vi "试剂余量显示UI.vi"() -> ()   [LabVIEW 2016, in "斯坦道氟化物.lvlib"]
uses:
  <vilib>/Utility/miscctls.llb/LVPointTypeDef.ctl
panel:
  in  "余量 14":string
  in  "余量 13":string
  in  "余量 12":string
  in  "余量 11":string
  in  "余量 10":string
  in  "余量 9":string
  in  "余量 8":string
  in  "余量 7":string
  in  "余量 6":string
  in  "余量 5":string
  in  "余量 4":string
  in  "余量 3":string
  in  "余量 2":string
  in  "余量":string
  in  "关闭":bool
  in  "全部重置":bool
  in  "试剂容量设置":bool
  in  "试剂名称设置":bool
  in  "重置 14":bool
  out "试剂 14":dbl(slide) caption="V9-2.试剂14" scale=0.0..100.0 scale format="%#_f %%"
  in  "重置 13":bool
  out "试剂 13":dbl(slide) caption="V9-1.试剂13" scale=0.0..100.0 scale format="%#_f %%"
  in  "重置 12":bool
  out "试剂 12":dbl(slide) caption="V12.试剂12" scale=0.0..100.0 scale format="%#_f %%"
  in  "重置 11":bool
  out "试剂 11":dbl(slide) caption="V11.试剂11" scale=0.0..100.0 scale format="%#_f %%"
  in  "重置 10":bool
  out "试剂 10":dbl(slide) caption="V10.试剂10" scale=0.0..100.0 scale format="%#_f %%"
  in  "重置 9":bool
  out "试剂 9":dbl(slide) caption="V9.试剂9" scale=0.0..100.0 scale format="%#_f %%"
  in  "重置 8":bool
  out "试剂 8":dbl(slide) caption="V8.试剂8" scale=0.0..100.0 scale format="%#_f %%"
  in  "重置 7":bool
  out "试剂 7":dbl(slide) caption="V7.试剂7" scale=0.0..100.0 scale format="%#_f %%"
  in  "重置 6":bool
  out "试剂 6":dbl(slide) caption="V6.试剂6" scale=0.0..100.0 scale format="%#_f %%"
  in  "重置 5":bool
  out "试剂 5":dbl(slide) caption="V5.试剂5" scale=0.0..100.0 scale format="%#_f %%"
  in  "重置 4":bool
  out "试剂 4":dbl(slide) caption="V4.试剂4" scale=0.0..100.0 scale format="%#_f %%"
  in  "重置 3":bool
  out "试剂 3":dbl(slide) caption="V3.试剂3" scale=0.0..100.0 scale format="%#_f %%"
  in  "重置 2":bool
  out "试剂 2":dbl(slide) caption="V2.试剂2" scale=0.0..100.0 scale format="%#_f %%"
  in  "重置":bool
  out "试剂":dbl(slide) caption="V1.试剂1" scale=0.0..100.0 scale format="%#_f %%"
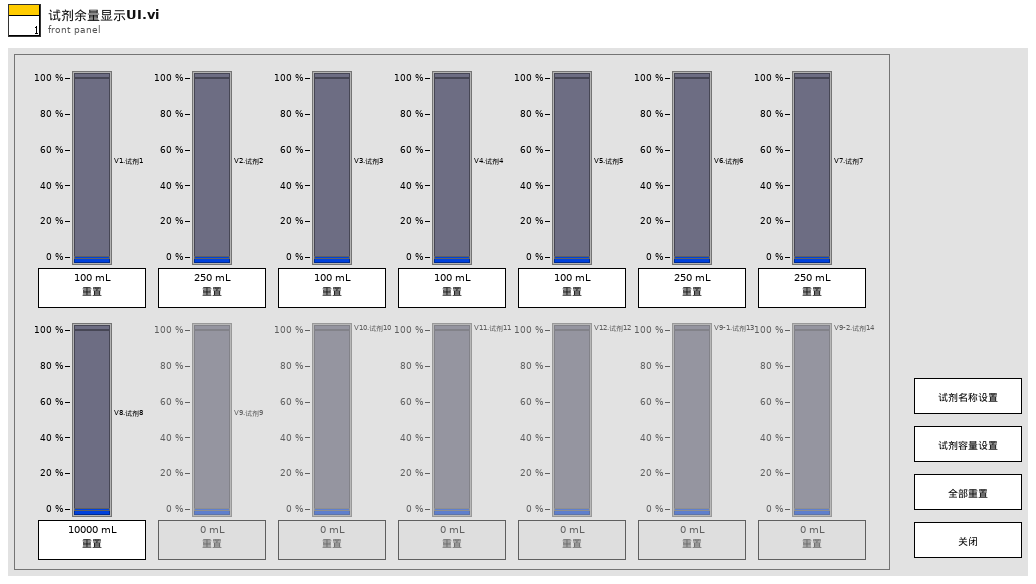
[diagram p1: front panel]
types:
  T1 = typedef "LVPointTypeDef.ctl" = cluster{"Horizontal":i16, "Vertical":i16}
  T2 = enum8{"Enabled", "Disabled", "Disabled and Grayed Out"}
  T3 = cluster{"时间标识":timestamp, "设备":string, "日志信息":string, "流程参数":string}
  T4 = cluster{"V1":sgl, "V2":sgl, "V3":sgl, "V4":sgl, "V5":sgl, "V6":sgl, "V7":sgl, "V8":sgl, "V9":sgl, "V10":sgl, "V11":sgl, "V12":sgl, "V9-1":sgl, "V9-2":sgl}
  T5 = cluster{"V":string, "V 2":string, "V 3":string, "V 4":string, "V 5":string, "V 6":string, "V 7":string, "V 8":string, "V 9":string, "V 10":string, "V 11":string, "V 12":string, "V9-1":string, "V9-2":string}
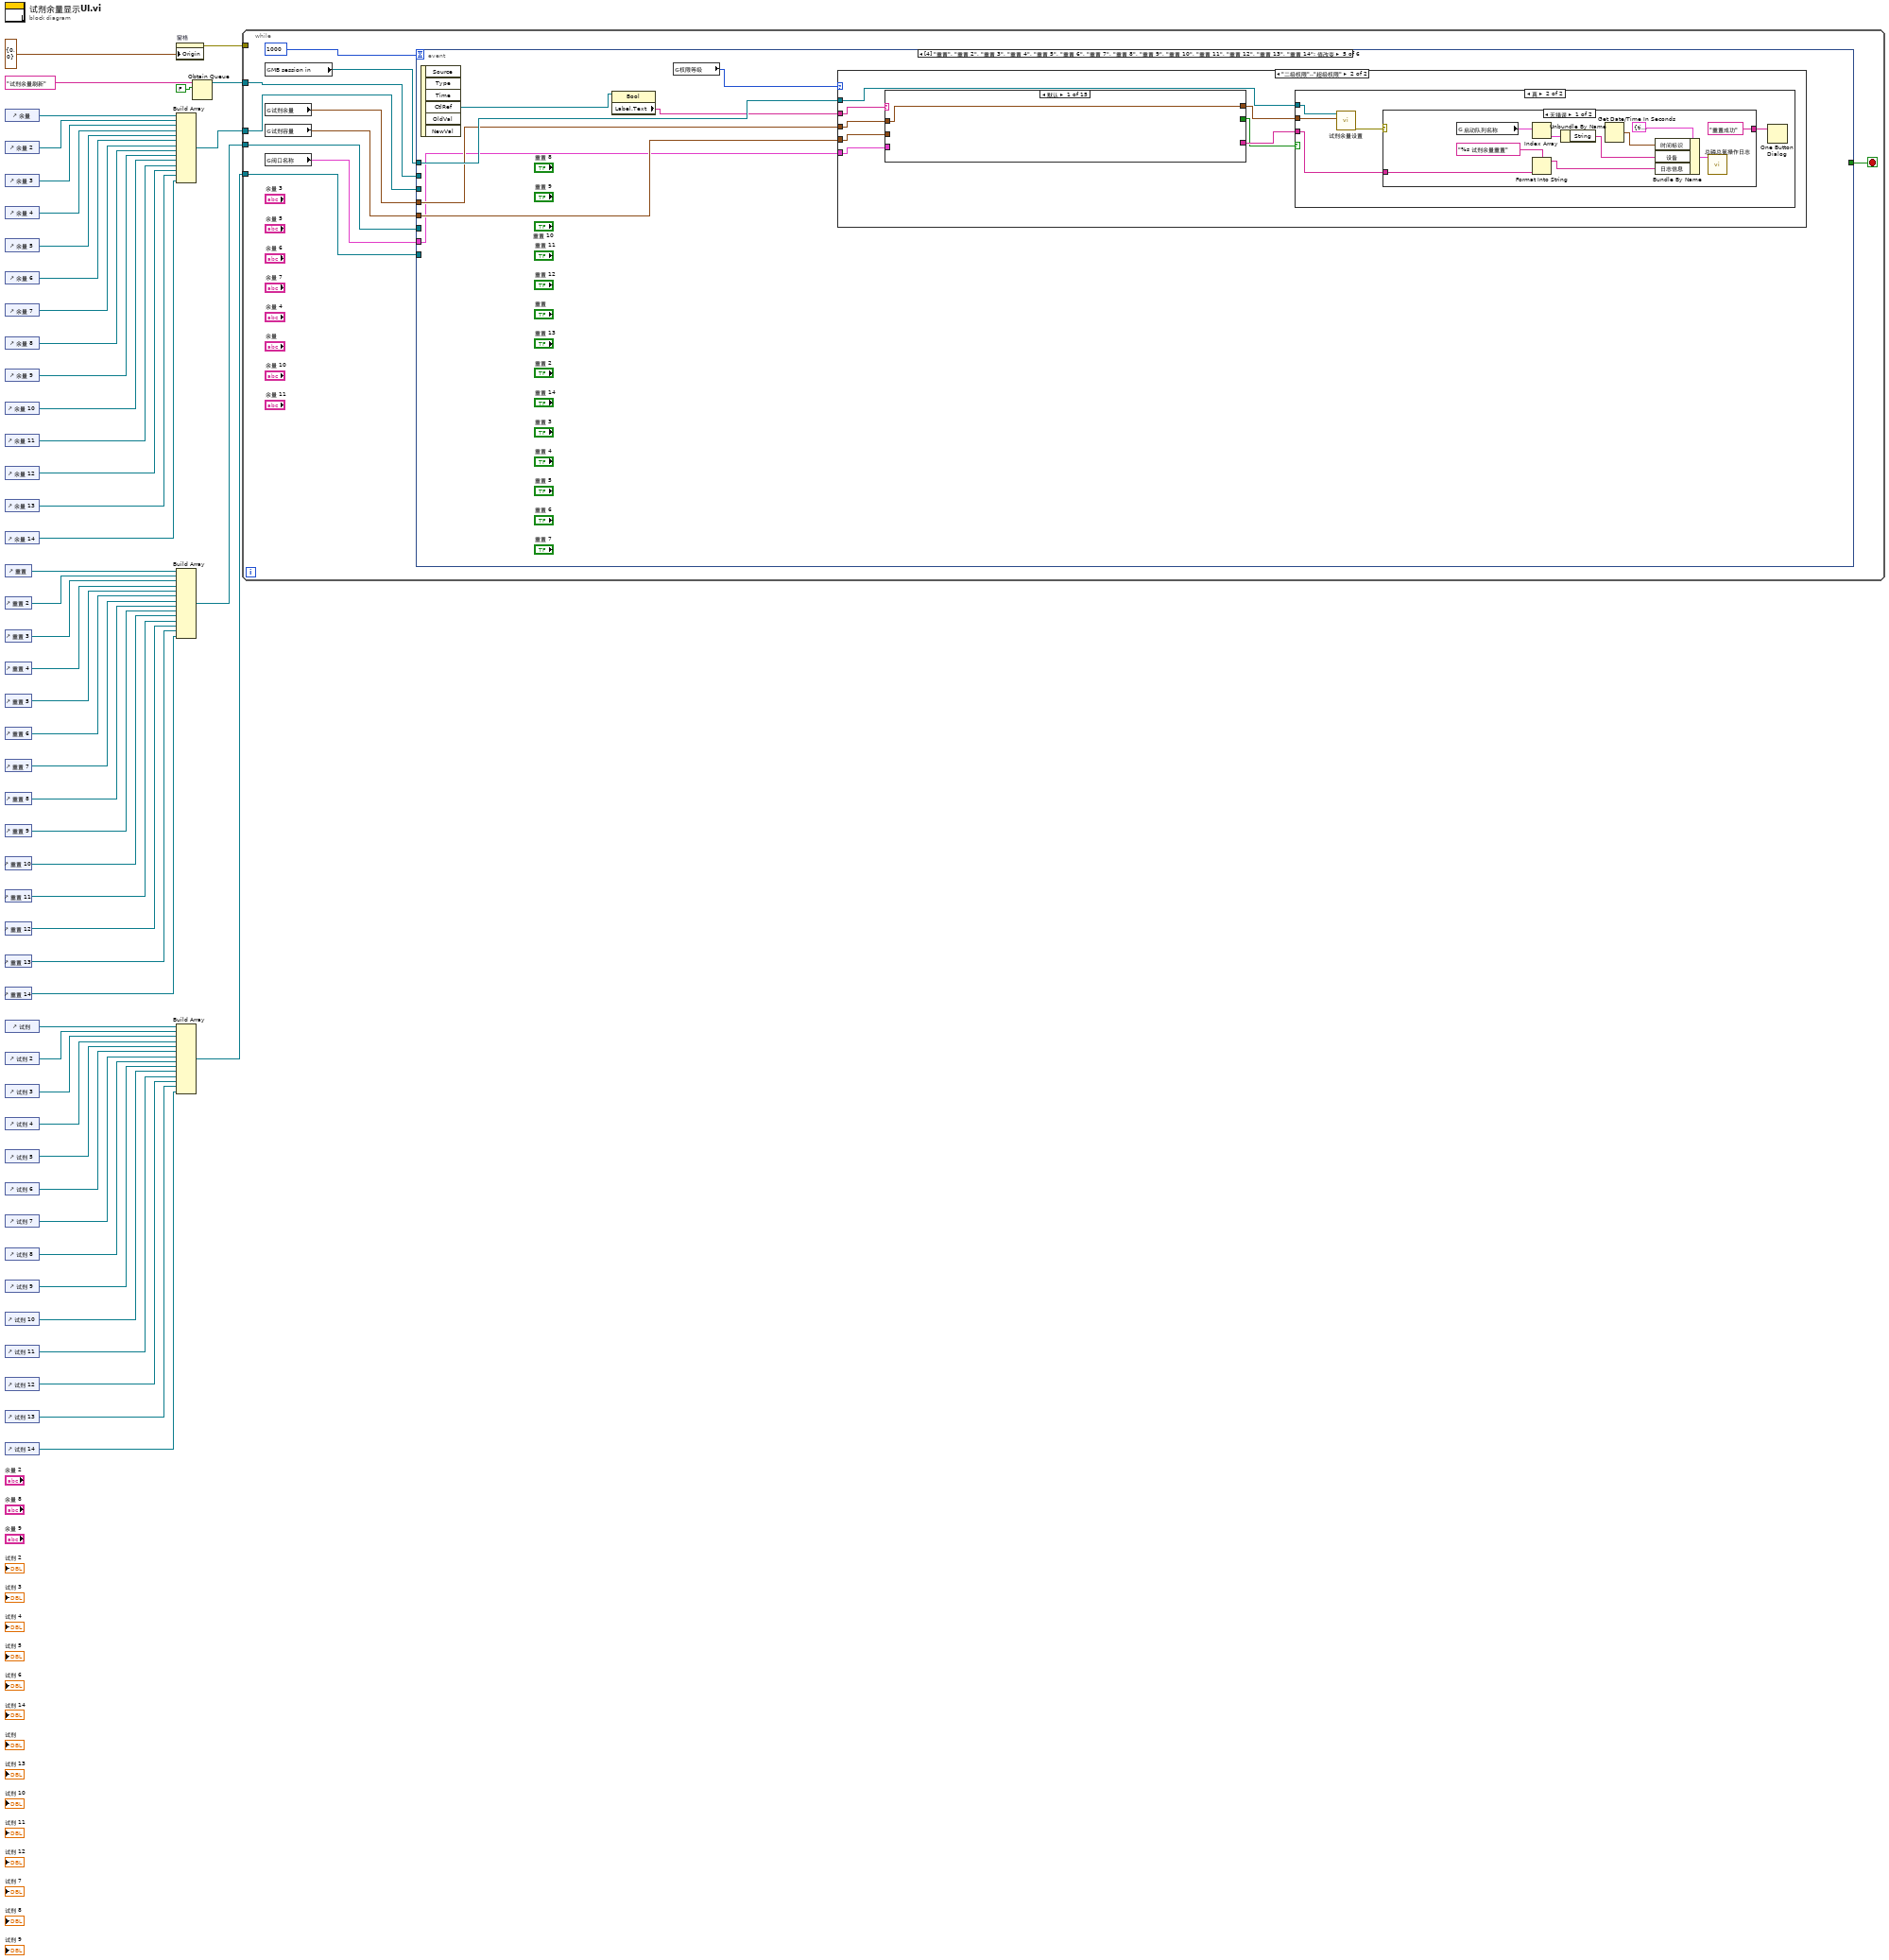
[diagram p0: block diagram]
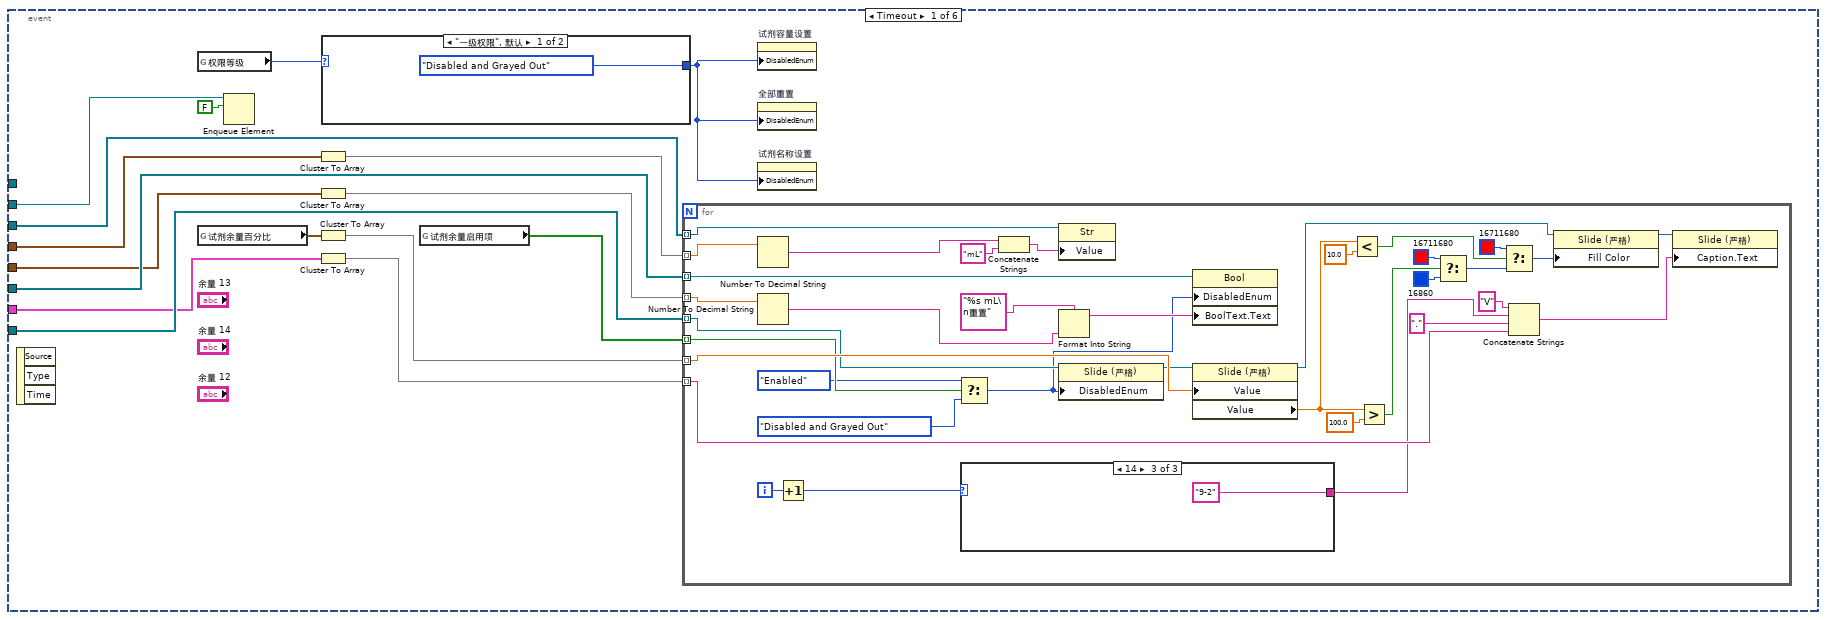
[diagram p2: hidden frame]
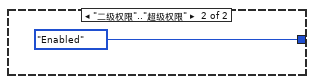
[diagram p3: hidden frame]
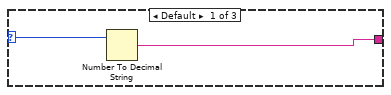
[diagram p4: hidden frame]
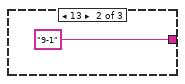
[diagram p5: hidden frame]
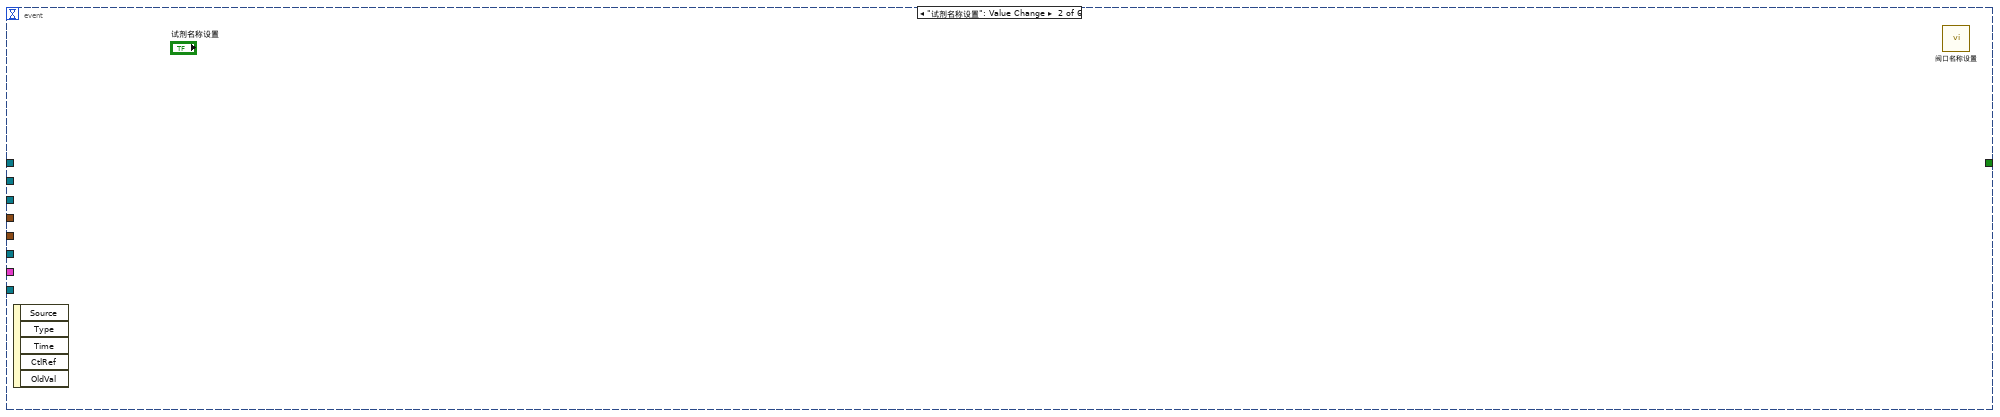
[diagram p6: hidden frame]
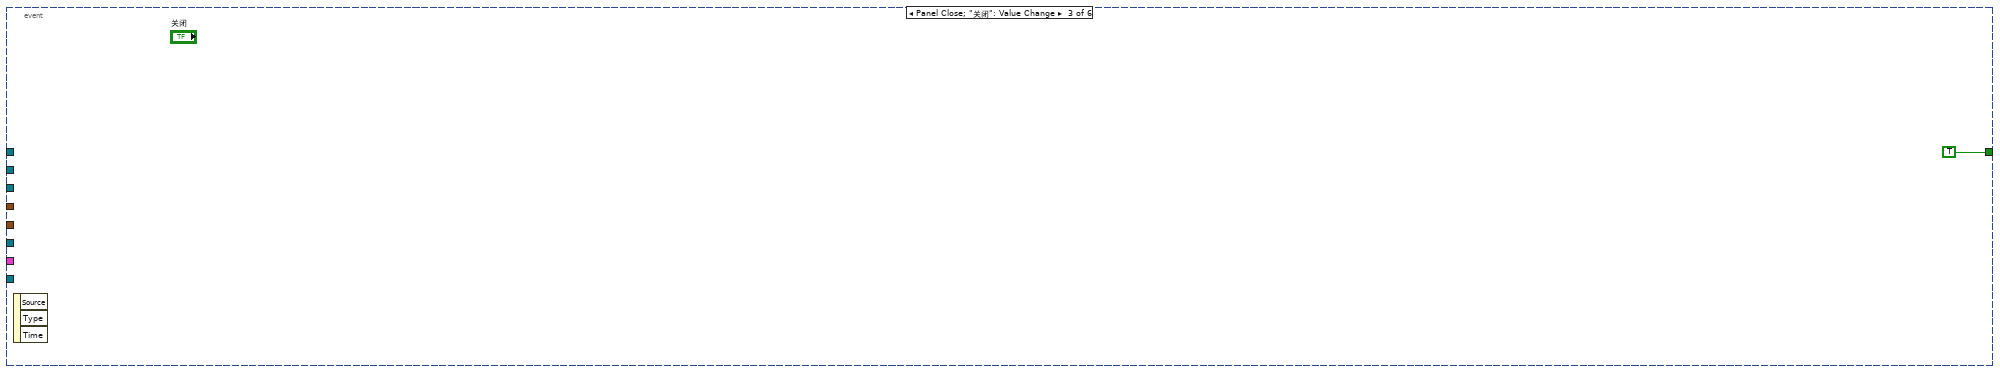
[diagram p7: hidden frame]
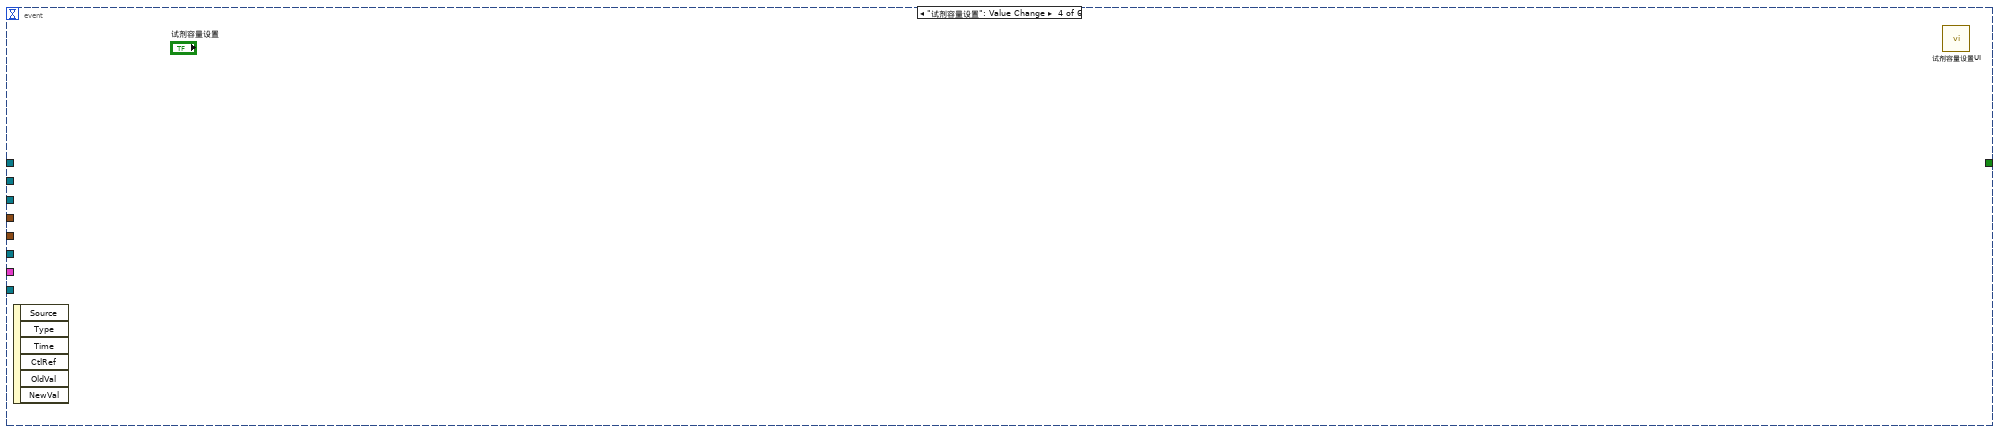
[diagram p8: hidden frame]
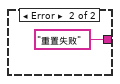
[diagram p11: hidden frame]
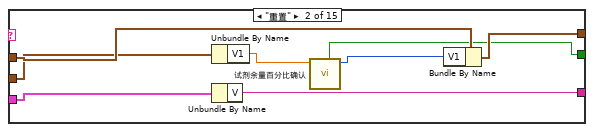
[diagram p12: hidden frame]
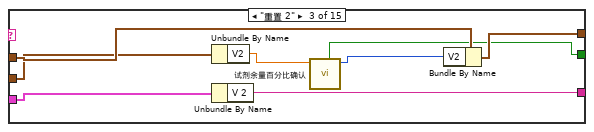
[diagram p13: hidden frame]
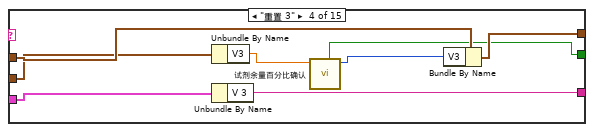
[diagram p14: hidden frame]
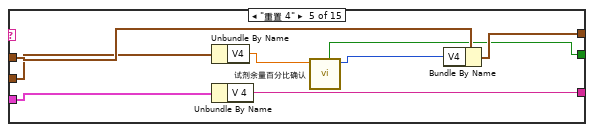
[diagram p15: hidden frame]
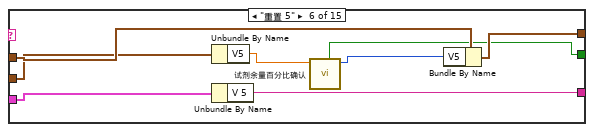
[diagram p16: hidden frame]
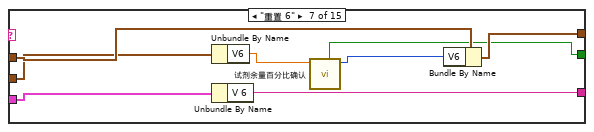
[diagram p17: hidden frame]
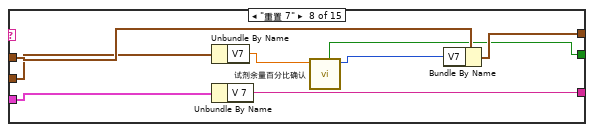
[diagram p18: hidden frame]
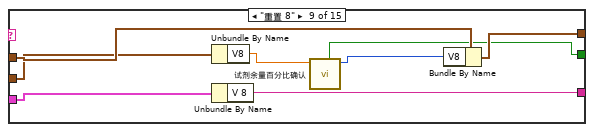
[diagram p19: hidden frame]
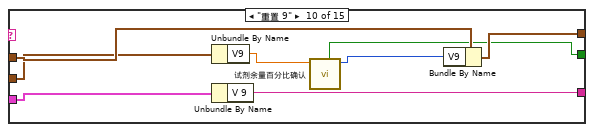
[diagram p20: hidden frame]
diagram:
  n1 = control-ref of="余量"() -> (w5:refnum<vi>)
  n2 = control-ref of="余量 2"() -> (w6:refnum<vi>)
  n3 = control-ref of="余量 3"() -> (w7:refnum<vi>)
  n4 = control-ref of="余量 4"() -> (w8:refnum<vi>)
  n5 = control-ref of="余量 5"() -> (w9:refnum<vi>)
  n6 = control-ref of="余量 6"() -> (w10:refnum<vi>)
  n7 = control-ref of="余量 7"() -> (w11:refnum<vi>)
  n8 = control-ref of="余量 8"() -> (w12:refnum<vi>)
  n9 = control-ref of="余量 9"() -> (w13:refnum<vi>)
  n10 = control-ref of="余量 10"() -> (w14:refnum<vi>)
  n11 = control-ref of="余量 11"() -> (w15:refnum<vi>)
  n12 = control-ref of="余量 12"() -> (w16:refnum<vi>)
  n13 = control-ref of="余量 13"() -> (w17:refnum<vi>)
  n14 = control-ref of="余量 14"() -> (w18:refnum<vi>)
  n15 = control-ref of="重置"() -> (w33:refnum<vi>)
  n16 = control-ref of="重置 2"() -> (w32:refnum<vi>)
  n17 = control-ref of="重置 3"() -> (w31:refnum<vi>)
  n18 = control-ref of="重置 4"() -> (w30:refnum<vi>)
  n19 = control-ref of="重置 5"() -> (w29:refnum<vi>)
  n20 = control-ref of="重置 6"() -> (w28:refnum<vi>)
  n21 = control-ref of="重置 7"() -> (w27:refnum<vi>)
  n22 = control-ref of="重置 8"() -> (w26:refnum<vi>)
  n23 = control-ref of="重置 9"() -> (w25:refnum<vi>)
  n24 = control-ref of="重置 10"() -> (w24:refnum<vi>)
  n25 = control-ref of="重置 11"() -> (w23:refnum<vi>)
  n26 = control-ref of="重置 12"() -> (w22:refnum<vi>)
  n27 = control-ref of="重置 13"() -> (w21:refnum<vi>)
  n28 = control-ref of="重置 14"() -> (w20:refnum<vi>)
  n29 = control-ref of="试剂"() -> (w50:refnum<vi>)
  n30 = control-ref of="试剂 2"() -> (w49:refnum<vi>)
  n31 = control-ref of="试剂 3"() -> (w48:refnum<vi>)
  n32 = control-ref of="试剂 4"() -> (w47:refnum<vi>)
  n33 = control-ref of="试剂 5"() -> (w46:refnum<vi>)
  n34 = control-ref of="试剂 6"() -> (w45:refnum<vi>)
  n35 = control-ref of="试剂 7"() -> (w44:refnum<vi>)
  n36 = control-ref of="试剂 8"() -> (w43:refnum<vi>)
  n37 = control-ref of="试剂 9"() -> (w42:refnum<vi>)
  n38 = control-ref of="试剂 10"() -> (w41:refnum<vi>)
  n39 = control-ref of="试剂 11"() -> (w40:refnum<vi>)
  n40 = control-ref of="试剂 12"() -> (w39:refnum<vi>)
  n41 = control-ref of="试剂 13"() -> (w38:refnum<vi>)
  n42 = control-ref of="试剂 14"() -> (w37:refnum<vi>)
  n43 = property on="窗格" class="Pane"("Origin"=T1 {"Horizontal"=0, "Vertical"=0} ("原点")) -> (error out=w34:errorcluster)  [unwired: 2 in, 1 out]
  n44 = Build Array(w5, w6, w7, w8, w9, w10, w11, w12, w13, w14, w15, w16, w17, w18) -> (w4:refnum<vi>[])
  n45 = Build Array(w33, w32, w31, w30, w29, w28, w27, w26, w25, w24, w23, w22, w21, w20) -> (w19:refnum<vi>[])
  n46 = Build Array(w50, w49, w48, w47, w46, w45, w44, w43, w42, w41, w40, w39, w38, w37) -> (w36:refnum<vi>[])
  n47 = Obtain Queue(name (unnamed)="试剂余量刷新" ("名称（未命名）"), element data type=FALSE) -> (queue out=w1:refnum<queue>)  [unwired: 3 in, 2 out]
  n48 = while {
    tunnel: w36 -> [w60]
    tunnel: w34 -> [_]
    tunnel: w19 -> [w59]
    tunnel: w4 -> [w55]
    tunnel: w1 -> [w51]
    stop <- w58 stop-if-true
    n49 = global read "VAR总磷总氮全局变量.vi" "MB session in"() -> (w56:refnum<class "MB_Master.lvclass">)
    n50 = global read "VAR总磷总氮全局变量.vi" "试剂余量"() -> (w53:T4)
    n51 = global read "VAR总磷总氮全局变量.vi" "试剂容量"() -> (w54:T4)
    n52 = global read "总磷总氮断电保存全局变量.vi" "阀口名称"() -> (w52:T5)
    n53 = event shown="[4] \"重置\", \"重置 2\", \"重置 3\", \"重置 4\", \"重置 5\", \"重置 6\", \"重置 7\", \"重置 8\", \"重置 9\", \"重置 10\", \"重置 11\", \"重置 12\", \"重置 13\", \"重置 14\": 值改变" {
      selector: _ -> [_ _ _ _ _ _]
      dyn-events: _ -> [_ _ _ _ _ _]
      timeout: 1000 -> [_ _ _ _ _ _]
      tunnel: w60 -> [w76 _ _ _ _ _]
      tunnel: w59 -> [w73 _ _ _ _ _]
      tunnel: [_ _ TRUE _ _ _] -> w58
      tunnel: w54 -> [w67 _ _ _ w122 _]
      tunnel: w53 -> [w66 _ _ _ w125 _]
      tunnel: w56 -> [_ _ _ _ w126 w265]
      tunnel: w55 -> [w70 _ _ _ _ _]
      tunnel: w52 -> [w63 _ _ _ w120 _]
      tunnel: w51 -> [w62 _ _ _ _ _]
      event Timeout {
        n54 = event-data() -> ()  [unwired: 1 in, 3 out]
        n55 = global read "VAR总磷总氮全局变量.vi" "权限等级"() -> (w65:enum16{"一级权限", "二级权限", "三级权限", "超级权限"})
        n56 = global read "VAR总磷总氮全局变量.vi" "试剂余量百分比"() -> (w68:T4)
        n57 = Enqueue Element(queue=w62, element=FALSE ("元素")) -> ()  [unwired: 2 in, 3 out]
        n58 = Cluster To Array(cluster=w66) -> (array=w71:sgl[])
        n59 = Cluster To Array(cluster=w67) -> (array=w74:sgl[])
        n60 = Cluster To Array(cluster=w68) -> (array=w75:sgl[])
        n61 = Cluster To Array(cluster=w63) -> (array=w72:string[])
        n62 = case shown="\"一级权限\", 默认" w65 {
          tunnel: [T2."Disabled and Grayed Out" ("禁用") T2."Enabled" ("禁用")] -> w64
          frame "一级权限", Default {
          }
          frame "二级权限".."超级权限" {
          }
        }
        n63 = global read "VAR总磷总氮全局变量.vi" "试剂余量启用项"() -> (w69:bool[])
        n64 = for {
          tunnel: w76 -> [w108] mode=indexing
          tunnel: w75 -> [w109] mode=indexing
          tunnel: w74 -> [w97] mode=indexing
          tunnel: w73 -> [w106] mode=indexing
          tunnel: w72 -> [w103] mode=indexing
          tunnel: w71 -> [w93] mode=indexing
          tunnel: w70 -> [w92] mode=indexing
          tunnel: w69 -> [w88] mode=indexing
          i -> [w100]
          n65 = Number To Decimal String(number=w93) -> (decimal integer string=w91:string)  [unwired: 1 in]
          n66 = Number To Decimal String(number=w97) -> (decimal integer string=w96:string)  [unwired: 1 in]
          n67 = Increment(x=w100) -> (x+1=w99:i32)
          n68 = Select(t=T2."Enabled" ("禁用"), s=w88, f=T2."Disabled and Grayed Out" ("禁用")) -> (s? t:f=w87:T2)
          n69 = case shown="14" w99 {
            selector: w99 -> [w116 _ _]
            tunnel: [w115 "9-1" "9-2"] -> w98
            frame Default {
              n70 = Number To Decimal String(number=w116) -> (decimal integer string=w115:string)  [unwired: 1 in]
            }
            frame 13 {
            }
            frame 14 {
            }
          }
          n71 = Concatenate Strings(w91, "mL" ("字符串")) -> (w90:string)
          n72 = property class="Str"(reference=w92, "Value"=w90) -> ()  [unwired: 1 in, 2 out]
          n73 = Format Into String(format string="%s mL\n重置" ("格式字符串"), w96) -> (resulting string=w94:string)  [unwired: 2 in, 1 out]
          n74 = property class="Slide (严格)"(reference=w108, "DisabledEnum"=w87) -> (reference out=w107:refnum<vi>)  [unwired: 1 in, 1 out]
          n75 = property class="Bool"(reference=w106, "DisabledEnum"=w87, "BoolText.Text"=w94) -> ()  [unwired: 1 in, 2 out]
          n76 = property class="Slide (严格)"(reference=w107, "Value"=w109) -> (reference out=w113:refnum<vi>, "Value"=w84:dbl)  [unwired: 1 in, 1 out]
          n77 = Less?(x=w84, y=10.0) -> (x < y?=w112:bool)
          n78 = Greater?(x=w84, y=100.0) -> (0:w82:bool)
          n79 = Select(t=u32 16711680 ("滑块颜色:背景色"), s=w82, f=u32 16860 ("滑块颜色:背景色")) -> (s? t:f=w79:u32)
          n80 = Select(t=u32 16711680 ("滑块颜色:背景色"), s=w112, f=w79) -> (s? t:f=w110:u32)
          n81 = Concatenate Strings("V" ("字符串"), w98, "." ("字符串"), w103) -> (w102:string)
          n82 = property class="Slide (严格)"(reference=w113, "Fill Color"=w110) -> (reference out=w105:refnum<vi>)  [unwired: 1 in, 1 out]
          n83 = property class="Slide (严格)"(reference=w105, "Caption.Text"=w102) -> ()  [unwired: 1 in, 2 out]
        }
        n84 = property on="试剂容量设置" class="Bool"("DisabledEnum"=w64) -> ()  [unwired: 2 in, 2 out]
        n85 = property on="全部重置" class="Bool"("DisabledEnum"=w64) -> ()  [unwired: 2 in, 2 out]
        n86 = property on="试剂名称设置" class="Bool"("DisabledEnum"=w64) -> ()  [unwired: 2 in, 2 out]
      }
      event "试剂名称设置": Value Change {
        n87 = event-data() -> ()  [unwired: 1 in, 5 out]
        n88 = call "阀口名称设置.vi"() -> ()  [unwired: 12 in]
      }
      event Panel Close; "关闭": Value Change {
        n89 = event-data() -> ()  [unwired: 1 in, 3 out]
      }
      event "试剂容量设置": Value Change {
        n90 = event-data() -> ()  [unwired: 1 in, 6 out]
        n91 = call "试剂容量设置UI.vi"() -> ()  [unwired: 12 in]
      }
      event "重置", "重置 2", "重置 3", "重置 4", "重置 5", "重置 6", "重置 7", "重置 8", "重置 9", "重置 10", "重置 11", "重置 12", "重置 13", "重置 14": Value Change {
        n92 = event-data() -> ("CtlRef"=w124:refnum<vi>)  [unwired: 1 in, 5 out]
        n93 = property class="Bool"(reference=w124) -> ("Label.Text"=w123:string)  [unwired: 1 in, 2 out]
        n94 = global read "VAR总磷总氮全局变量.vi" "权限等级"() -> (w121:enum16{"一级权限", "二级权限", "三级权限", "超级权限"})
        n95 = case shown="\"二级权限\"..\"超级权限\"" w121 {
          tunnel: w126 -> [_ w134]
          tunnel: w125 -> [_ w133]
          tunnel: w123 -> [_ w131]
          tunnel: w122 -> [_ w130]
          tunnel: w120 -> [_ w129]
          frame "一级权限", Default {
          }
          frame "二级权限".."超级权限" {
            n96 = case shown="默认" w131 {
              tunnel: w133 -> [w151 w159 w167 w175 w183 w191 w199 w207 w215 w223 w231 w239 w247 w255 w263]
              tunnel: [w151 w158 w166 w174 w182 w190 w198 w206 w214 w222 w230 w238 w246 w254 w262] -> w132
              tunnel: w130 -> [_ w157 w165 w173 w181 w189 w197 w205 w213 w221 w229 w237 w245 w253 w261]
              tunnel: w129 -> [_ w154 w162 w170 w178 w186 w194 w202 w210 w218 w226 w234 w242 w250 w258]
              tunnel: [_ w153 w161 w169 w177 w185 w193 w201 w209 w217 w225 w233 w241 w249 w257] -> w128
              tunnel: [_ w152 w160 w168 w176 w184 w192 w200 w208 w216 w224 w232 w240 w248 w256] -> w127
              frame Default {
              }
              frame "重置" {
                n97 = Unbundle By Name(w157) -> ("V1"=w156:sgl)
                n98 = Unbundle By Name(w154) -> ("V"=w153:string)
                n99 = call "试剂余量百分比确认.vi"("试剂余量百分比 2"=w156) -> ("Value"=w155:u16, "check ？"=w152:bool)  [unwired: 9 in]
                n100 = Bundle By Name(cluster=w159, "V1"=w155) -> (w158:T4)
              }
              frame "重置 2" {
                n101 = Unbundle By Name(w165) -> ("V2"=w164:sgl)
                n102 = Unbundle By Name(w162) -> ("V 2"=w161:string)
                n103 = call "试剂余量百分比确认.vi"("试剂余量百分比 2"=w164) -> ("Value"=w163:u16, "check ？"=w160:bool)  [unwired: 9 in]
                n104 = Bundle By Name(cluster=w167, "V2"=w163) -> (w166:T4)
              }
              frame "重置 3" {
                n105 = Unbundle By Name(w173) -> ("V3"=w172:sgl)
                n106 = Unbundle By Name(w170) -> ("V 3"=w169:string)
                n107 = call "试剂余量百分比确认.vi"("试剂余量百分比 2"=w172) -> ("Value"=w171:u16, "check ？"=w168:bool)  [unwired: 9 in]
                n108 = Bundle By Name(cluster=w175, "V3"=w171) -> (w174:T4)
              }
              frame "重置 4" {
                n109 = Unbundle By Name(w181) -> ("V4"=w180:sgl)
                n110 = Unbundle By Name(w178) -> ("V 4"=w177:string)
                n111 = call "试剂余量百分比确认.vi"("试剂余量百分比 2"=w180) -> ("Value"=w179:u16, "check ？"=w176:bool)  [unwired: 9 in]
                n112 = Bundle By Name(cluster=w183, "V4"=w179) -> (w182:T4)
              }
              frame "重置 5" {
                n113 = Unbundle By Name(w189) -> ("V5"=w188:sgl)
                n114 = Unbundle By Name(w186) -> ("V 5"=w185:string)
                n115 = call "试剂余量百分比确认.vi"("试剂余量百分比 2"=w188) -> ("Value"=w187:u16, "check ？"=w184:bool)  [unwired: 9 in]
                n116 = Bundle By Name(cluster=w191, "V5"=w187) -> (w190:T4)
              }
              frame "重置 6" {
                n117 = Unbundle By Name(w197) -> ("V6"=w196:sgl)
                n118 = Unbundle By Name(w194) -> ("V 6"=w193:string)
                n119 = call "试剂余量百分比确认.vi"("试剂余量百分比 2"=w196) -> ("Value"=w195:u16, "check ？"=w192:bool)  [unwired: 9 in]
                n120 = Bundle By Name(cluster=w199, "V6"=w195) -> (w198:T4)
              }
              frame "重置 7" {
                n121 = Unbundle By Name(w205) -> ("V7"=w204:sgl)
                n122 = Unbundle By Name(w202) -> ("V 7"=w201:string)
                n123 = call "试剂余量百分比确认.vi"("试剂余量百分比 2"=w204) -> ("Value"=w203:u16, "check ？"=w200:bool)  [unwired: 9 in]
                n124 = Bundle By Name(cluster=w207, "V7"=w203) -> (w206:T4)
              }
              frame "重置 8" {
                n125 = Unbundle By Name(w213) -> ("V8"=w212:sgl)
                n126 = Unbundle By Name(w210) -> ("V 8"=w209:string)
                n127 = call "试剂余量百分比确认.vi"("试剂余量百分比 2"=w212) -> ("Value"=w211:u16, "check ？"=w208:bool)  [unwired: 9 in]
                n128 = Bundle By Name(cluster=w215, "V8"=w211) -> (w214:T4)
              }
              frame "重置 9" {
                n129 = Unbundle By Name(w221) -> ("V9"=w220:sgl)
                n130 = Unbundle By Name(w218) -> ("V 9"=w217:string)
                n131 = call "试剂余量百分比确认.vi"("试剂余量百分比 2"=w220) -> ("Value"=w219:u16, "check ？"=w216:bool)  [unwired: 9 in]
                n132 = Bundle By Name(cluster=w223, "V9"=w219) -> (w222:T4)
              }
              frame "重置 10" {
                n133 = Unbundle By Name(w229) -> ("V10"=w228:sgl)
                n134 = Unbundle By Name(w226) -> ("V 10"=w225:string)
                n135 = call "试剂余量百分比确认.vi"("试剂余量百分比 2"=w228) -> ("Value"=w227:u16, "check ？"=w224:bool)  [unwired: 9 in]
                n136 = Bundle By Name(cluster=w231, "V10"=w227) -> (w230:T4)
              }
              frame "重置 11" {
                n137 = Unbundle By Name(w237) -> ("V11"=w236:sgl)
                n138 = Unbundle By Name(w234) -> ("V 11"=w233:string)
                n139 = call "试剂余量百分比确认.vi"("试剂余量百分比 2"=w236) -> ("Value"=w235:u16, "check ？"=w232:bool)  [unwired: 9 in]
                n140 = Bundle By Name(cluster=w239, "V11"=w235) -> (w238:T4)
              }
              frame "重置 12" {
                n141 = Unbundle By Name(w245) -> ("V12"=w244:sgl)
                n142 = Unbundle By Name(w242) -> ("V 12"=w241:string)
                n143 = call "试剂余量百分比确认.vi"("试剂余量百分比 2"=w244) -> ("Value"=w243:u16, "check ？"=w240:bool)  [unwired: 9 in]
                n144 = Bundle By Name(cluster=w247, "V12"=w243) -> (w246:T4)
              }
              frame "重置 13" {
                n145 = Unbundle By Name(w253) -> ("V9-1"=w252:sgl)
                n146 = Unbundle By Name(w250) -> ("V9-1"=w249:string)
                n147 = call "试剂余量百分比确认.vi"("试剂余量百分比 2"=w252) -> ("Value"=w251:u16, "check ？"=w248:bool)  [unwired: 9 in]
                n148 = Bundle By Name(cluster=w255, "V9-1"=w251) -> (w254:T4)
              }
              frame "重置 14" {
                n149 = Unbundle By Name(w261) -> ("V9-2"=w260:sgl)
                n150 = Unbundle By Name(w258) -> ("V9-2"=w257:string)
                n151 = call "试剂余量百分比确认.vi"("试剂余量百分比 2"=w260) -> ("Value"=w259:u16, "check ？"=w256:bool)  [unwired: 9 in]
                n152 = Bundle By Name(cluster=w263, "V9-2"=w259) -> (w262:T4)
              }
            }
            n153 = case shown="真" w127 {
              tunnel: w134 -> [_ w139]
              tunnel: w132 -> [_ w138]
              tunnel: w128 -> [_ w135]
              frame False {
              }
              frame True {
                n154 = call "试剂余量设置.vi"("试剂余量"=w138, "MB session in"=w139) -> ("error out"=w137:errorcluster)  [unwired: 8 in, 1 out]
                n155 = case shown="无错误" w137 {
                  tunnel: ["重置成功" ("消息") "重置失败" ("消息")] -> w136
                  tunnel: w135 -> [w142 _]
                  frame No Error {
                    n156 = global read "model config var.vi" "启动队列名称"() -> (w146:cluster{"String":string, "Value":u16}[])
                    n157 = Index Array(array=w146) -> (element=w147:cluster{"String":string, "Value":u16})  [unwired: 1 in]
                    n158 = Format Into String(format string="%s 试剂余量重置" ("格式字符串"), w142) -> (resulting string=w140:string)  [unwired: 2 in, 1 out]
                    n159 = Unbundle By Name(w147) -> ("String"=w148:string)
                    n160 = Get Date/Time In Seconds() -> (seconds since 1Jan1904=w145:timestamp)
                    n161 = Bundle By Name(cluster=T3 {"时间标识"=timestamp(0 s since 1904-01-01), "设备"="", "日志信息"="", "流程参数"=""} ("data in"), "时间标识"=w145, "设备"=w148, "日志信息"=w140) -> (w144:T3)
                    n162 = call "总磷总氮操作日志.vi"("data in"=w144) -> ()  [unwired: 10 in, 1 out]
                  }
                  frame Error {
                  }
                }
                n163 = One Button Dialog(message=w136) -> ()  [unwired: 1 in, 1 out]
              }
            }
          }
        }
      }
      event "全部重置": Value Change {
        n164 = event-data() -> ()  [unwired: 1 in, 6 out]
        n165 = global read "VAR总磷总氮全局变量.vi" "权限等级"() -> (w264:enum16{"一级权限", "二级权限", "三级权限", "超级权限"})
        n166 = case shown="\"二级权限\"..\"超级权限\"" w264 {
          tunnel: w265 -> [_ w268]
          frame "一级权限", Default {
          }
          frame "二级权限".."超级权限" {
            n167 = call "试剂余量重置.vi"("MB session in"=w268) -> ("error out"=w266:errorcluster)  [unwired: 9 in, 1 out]
            n168 = case shown="错误" w266 {
              tunnel: ["重置成功" ("消息") "重置失败" ("消息")] -> w267
              frame No Error {
              }
              frame Error {
              }
            }
            n169 = One Button Dialog(message=w267) -> ()  [unwired: 1 in, 1 out]
          }
        }
      }
    }
  }
